vi "Tags Dialog.vi"(8 "error in (no error)":errorcluster, 11 "Tag Data In":T1[](array[typedef])) -> (0 "error out":errorcluster, 1 "Cancelled?":bool=TRUE, 2 "UI Refresh Needed?":bool, 3 "Tag Data Out":T1[](array[typedef]))   [LabVIEW 2018, in "OPC UA.lvlib"]
uses:
  OPC Tag Data.ctl
  <vilib>/Utility/xml.llb/Write to XML File(string).vi
  OPC UA.lvlib
  Settings/Settings.lvlib
panel:
  in  "Tag Data":T2(array[cluster])
  in  "Cancel Button":bool
  in  "OK Button":bool
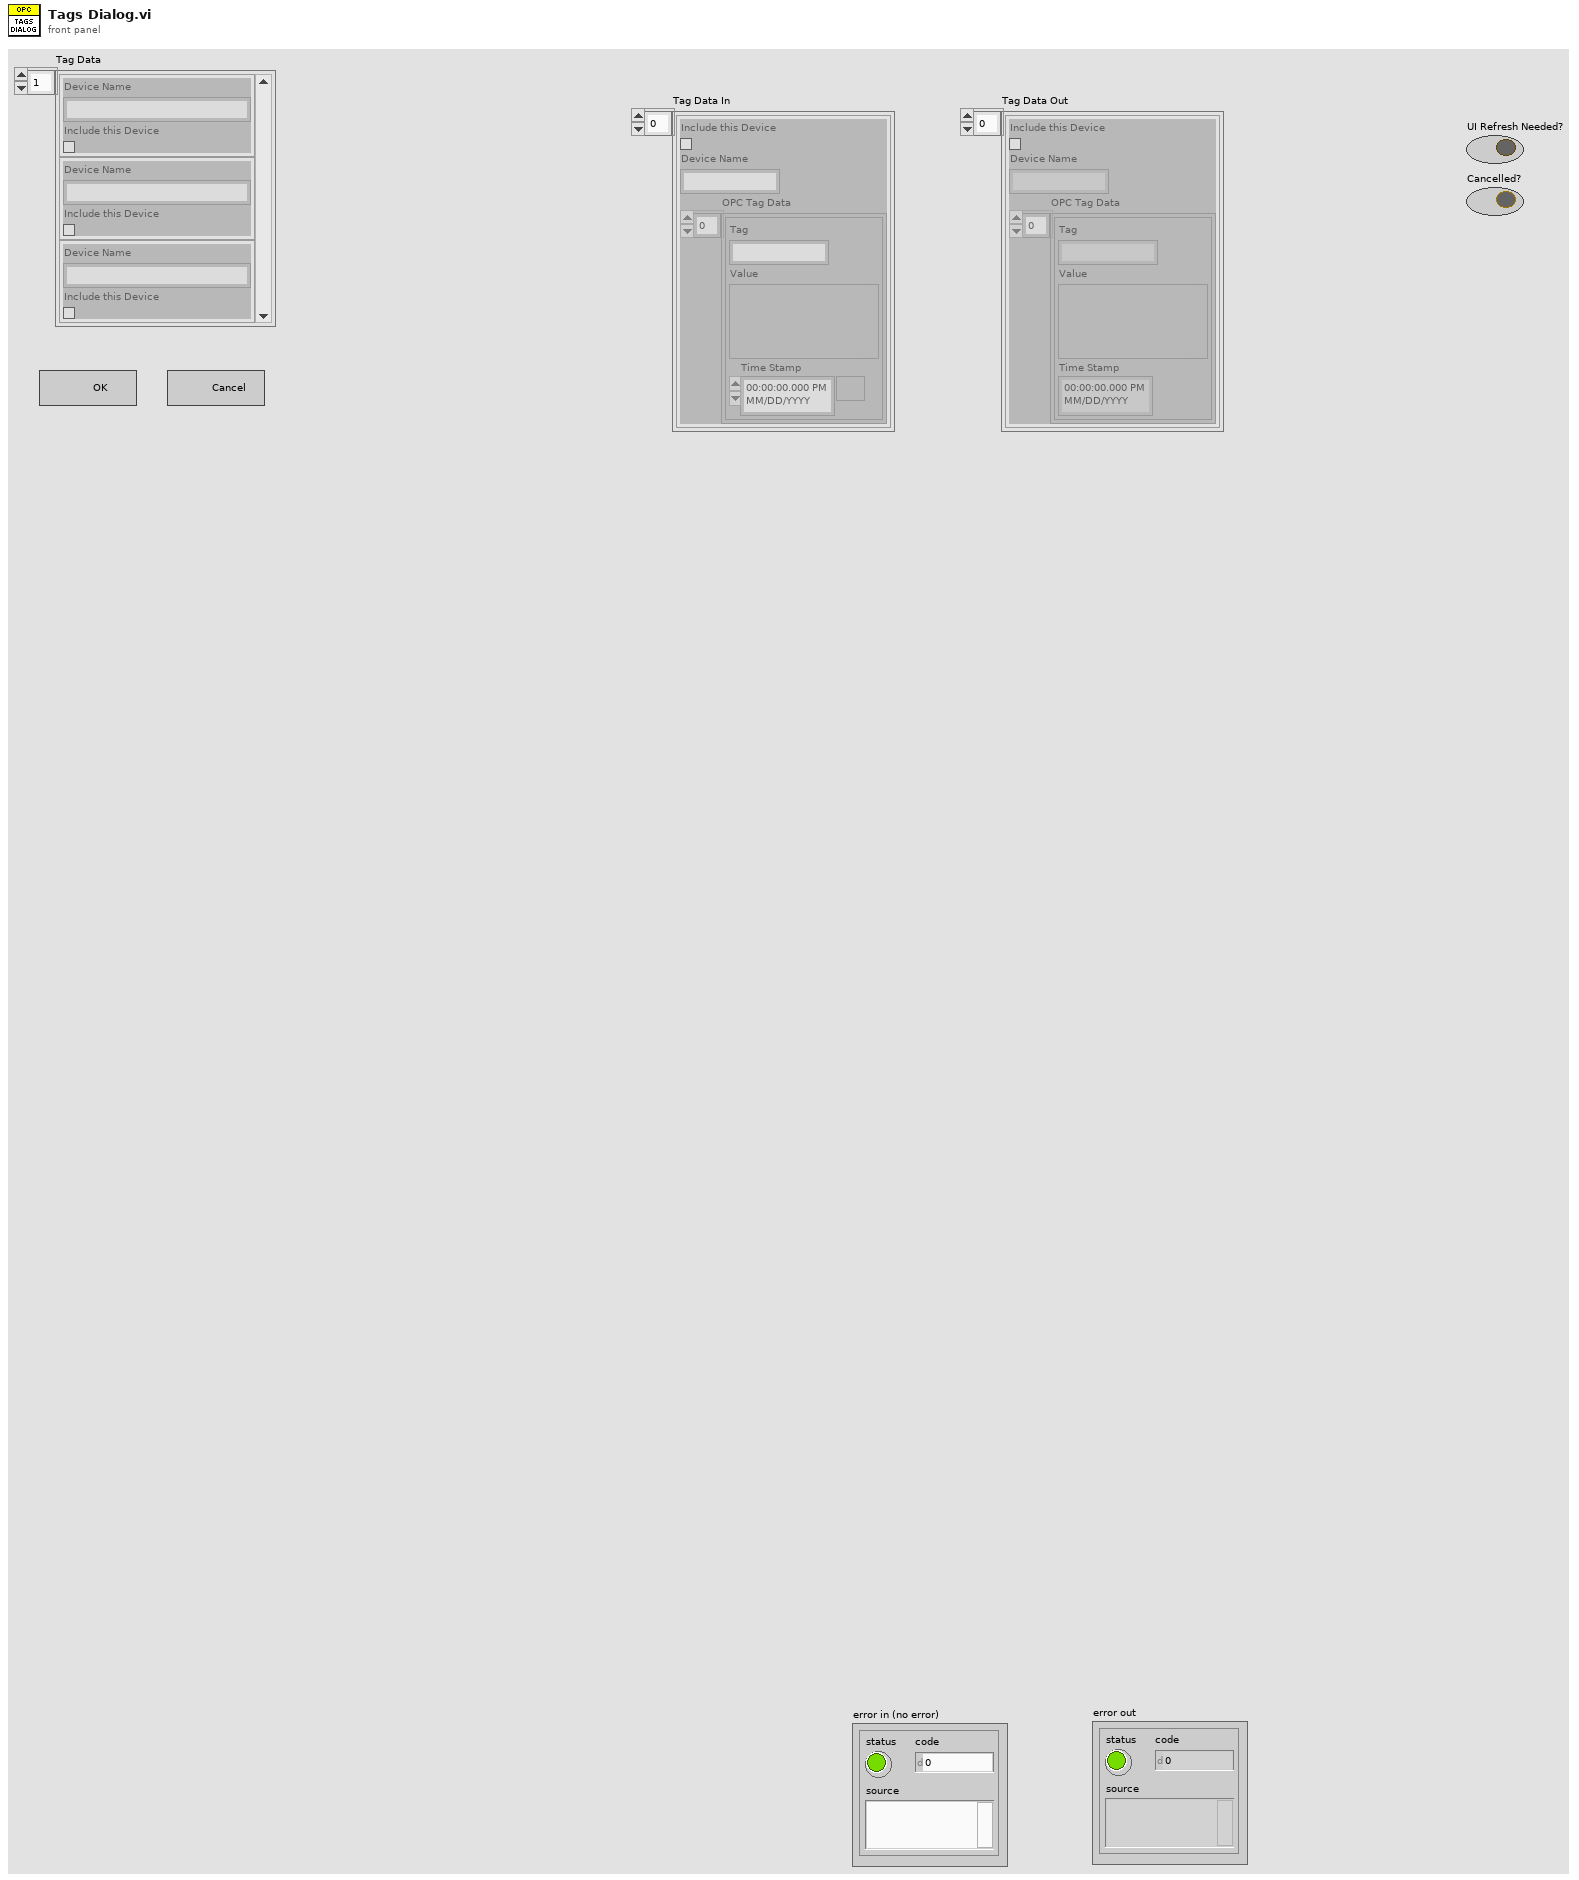
[diagram p1: front panel]
types:
  T1 = typedef "OPC UA.lvlib/OPC Tag Data.ctl" = cluster{"Include this Device":bool, "Device Name":string, "OPC Tag Data":cluster{"Tag":string, "Value":variant, "Time Stamp":timestamp}[]}
  T2 = cluster{"Device Name":string, "Include this Device":bool}[]
  T3 = cluster{"Device Name":string, "Include this Device":bool}
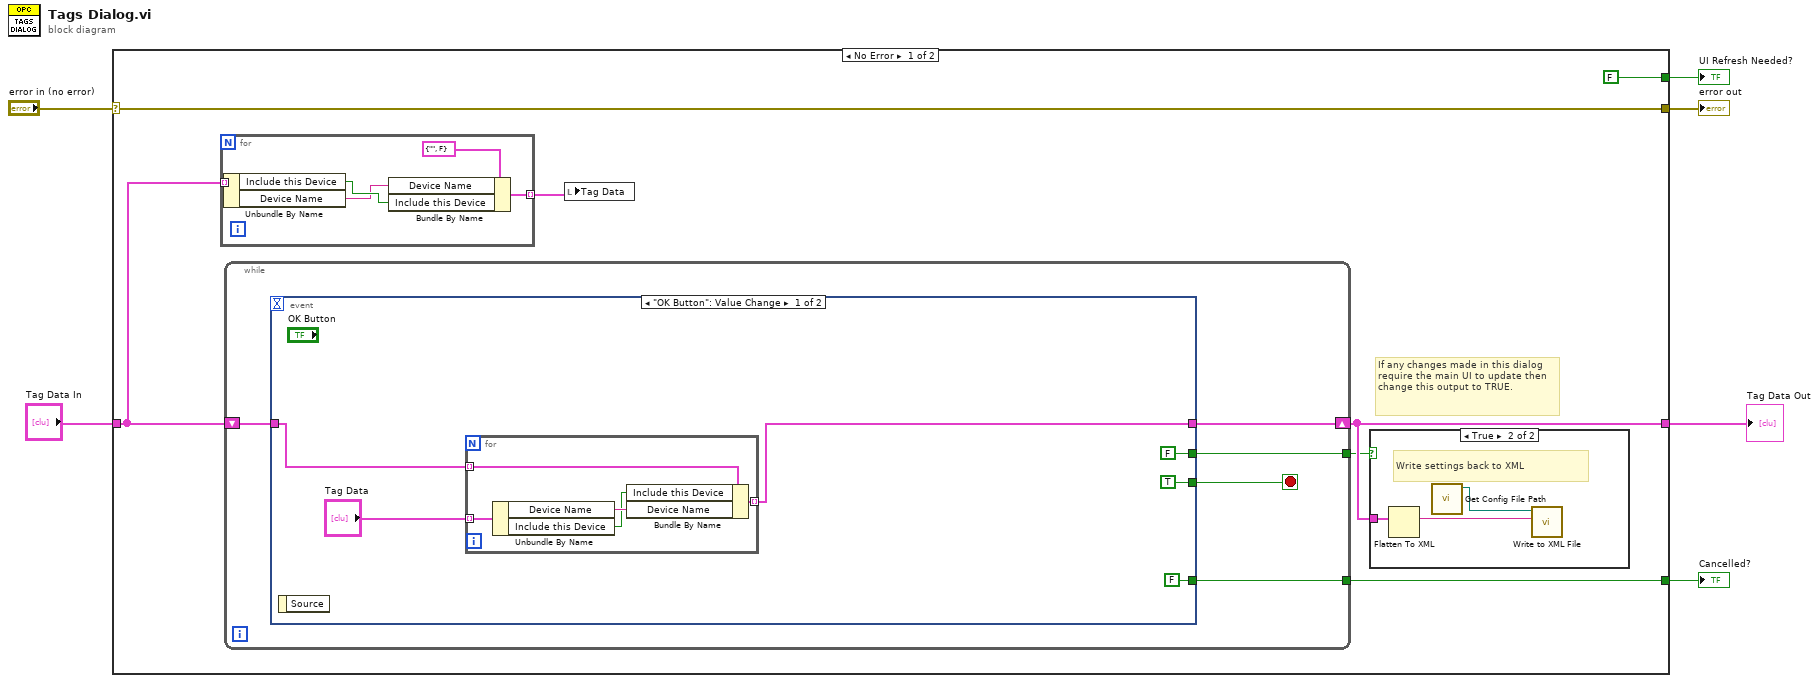
[diagram p0: block diagram]
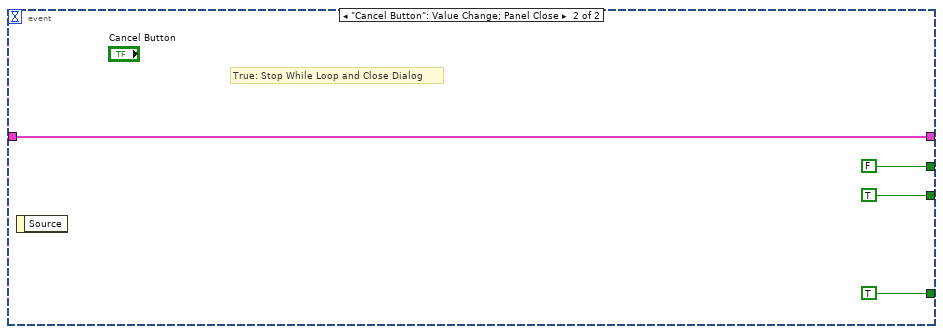
[diagram p2: hidden frame]
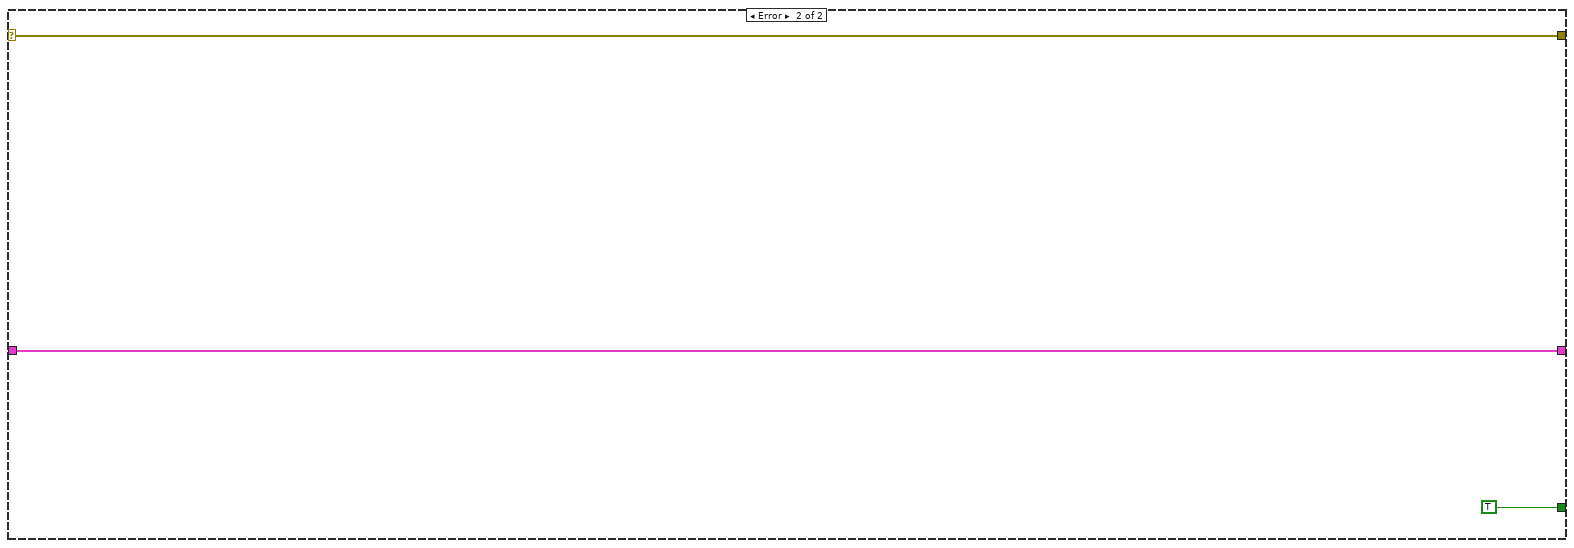
[diagram p4: hidden frame]
diagram:
  n1 = case shown="No Error" "error in (no error)" {
    selector: "error in (no error)" -> [w13 w44]
    tunnel: [w13 w44] -> w6
    tunnel: "Tag Data In" -> [w8 w43]
    tunnel: [w11 w43] -> w1
    tunnel: [FALSE ("UI Refresh Needed?") _] -> w5
    tunnel: [w9 TRUE ("UI Refresh Needed?")] -> w4
    frame No Error {
      # "If any changes made in this dialog require the main UI to update then change this output to TRUE."
      n2 = for {
        tunnel: w8 -> [w18] mode=indexing
        tunnel: [w15] -> w7 mode=indexing
        n3 = Unbundle By Name(w18) -> ("Include this Device"=w17:bool, "Device Name"=w16:string)
        n4 = Bundle By Name(cluster=T3 {"Device Name"="", "Include this Device"=FALSE}, "Device Name"=w16, "Include this Device"=w17) -> (w15:T3)
      }
      n5 = while {
        tunnel: [w23] -> w10
        tunnel: [w20] -> w9
        shift-right: [w22] -> w11
        shift-left: w8 -> [w19]
        stop <- w21 stop-if-true
        n6 = event shown="[0] \"OK Button\": Value Change" {
          selector: _ -> [_ _]
          dyn-events: _ -> [_ _]
          timeout: _ -> [_ _]
          tunnel: [w24 w38] -> w22
          tunnel: w19 -> [w25 w38]
          tunnel: [FALSE ("UI Refresh Needed?") FALSE ("UI Refresh Needed?")] -> w23
          tunnel: [TRUE TRUE] -> w21
          tunnel: [FALSE ("UI Refresh Needed?") TRUE ("UI Refresh Needed?")] -> w20
          event "OK Button": Value Change {
            n7 = event-data() -> ()  [unwired: 1 in, 1 out]
            n8 = for {
              tunnel: "Tag Data" -> [w33] mode=indexing
              tunnel: w25 -> [w34] mode=indexing
              tunnel: [w30] -> w24 mode=indexing
              n9 = Unbundle By Name(w33) -> ("Device Name"=w32:string, "Include this Device"=w31:bool)
              n10 = Bundle By Name(cluster=w34, "Include this Device"=w31, "Device Name"=w32) -> (w30:T1)
            }
          }
          event "Cancel Button": Value Change; Panel Close {
            # "True: Stop While Loop and Close Dialog"
            n11 = event-data() -> ()  [unwired: 1 in, 1 out]
          }
        }
      }
      n12 = local write "Tag Data"(w7) -> ()
      n13 = case shown="True" w10 {
        tunnel: w11 -> [_ w40]
        frame False {
        }
        frame True {
          # "Write settings back to XML"
          n14 = Flatten To XML(anything=w40) -> (xml string=w39:string)
          n15 = call "Get Config File Path.vi"() -> ("XML File Path"=w41:path)  [unwired: 10 in, 1 out]
          n16 = call-poly <vilib>:"Write to XML File.vi"("XML Input"=w39, "XML File Path"=w41) -> ()  [unwired: 7 in, 3 out]
        }
      }
    }
    frame Error {
    }
  }
  "UI Refresh Needed?" <- w5
  "error out" <- w6
  "Cancelled?" <- w4
  "Tag Data Out" <- w1
